vi "Close XL WorkBook.vi"(8 "error in":errorcluster, 9 "Workbook":T1, 10 "Excel._Workbook":refnum<k7>, 11 "Excel._Application":refnum<k7>) -> (0 "error out":errorcluster, 3 "Excel._Application":refnum<k7>)   [LabVIEW 2017]
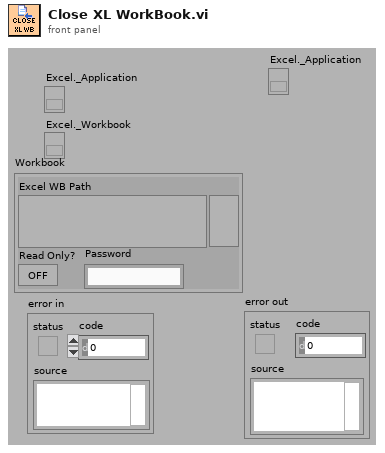
[diagram p1: front panel]
types:
  T1 = cluster{"Excel WB Path":path, "Read Only?":bool, "Password":string}
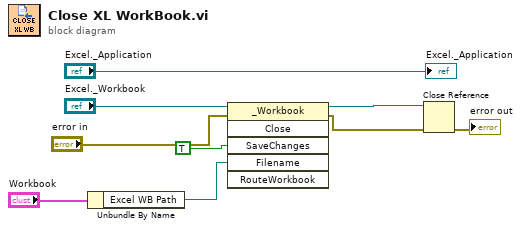
[diagram p0: block diagram]
diagram:
  n1 = Unbundle By Name("Workbook") -> ("Excel WB Path"=w4:path)
  n2 = invoke class="_Workbook" method="Close"(reference="Excel._Workbook", error in="error in", "SaveChanges"=TRUE, "Filename"=w4) -> (reference out=w6:refnum<k7>, error out=w1:errorcluster)  [unwired: 2 in, 4 out]
  n3 = Close Reference(reference=w6, error in (no error)=w1) -> (error out=→"error out":errorcluster)
  "Excel._Application" <- "Excel._Application"
